vi "Read latest Position.vi"(8 "error in (no error)":errorcluster, 11 "FINE SIM Motion Axis":refnum<class "FINE SIM Motion Axis.lvclass">) -> (0 "error out":errorcluster, 2 "Current Position":dbl, 3 "FINE SIM Motion Axis":refnum<class "FINE SIM Motion Axis.lvclass">)   [LabVIEW 2022 SP3, in "FINE SIM Motion Axis.lvclass"]
uses:
  FINE SIM Motion Axis.lvclass
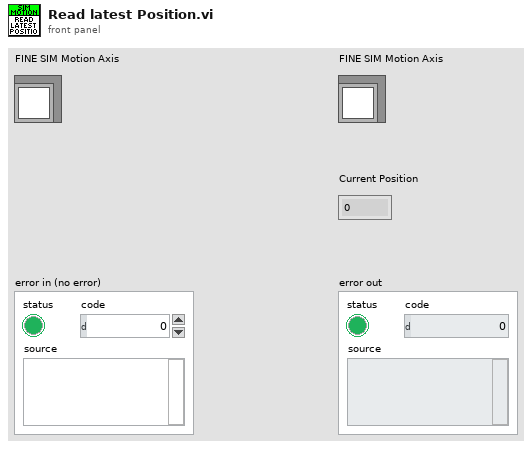
[diagram p1: front panel]
types:
  T1 = typedef "FINE SIM Motion Axis.lvclass/Axis Data.ctl" = cluster{"Axis Parameters":T2, "Time Stamp":timestamp, "Settings":T4}
  T2 = typedef "FINE SIM Motion Axis.lvclass/Axis Parameters.ctl" = cluster{"Moving":bool, "Homed":bool, "Desired Position":dbl, "Current Positon":dbl, "Current Speed":dbl, "Home Status":T3}
  T3 = typedef "FINE SIM Motion Axis.lvclass/Homing Status.ctl" = enum16{"Idle", "Inital Home Motion", "Final Home Motion", "Done Homing"}
  T4 = typedef "FINE SIM Motion Axis.lvclass/Settings.ctl" = cluster{"Axis Name":string, "Axis Settings":T5}
  T5 = typedef "FINE SIM Motion Axis.lvclass/Axis Settings.ctl" = cluster{"Speed":dbl, "Acceleration":dbl}
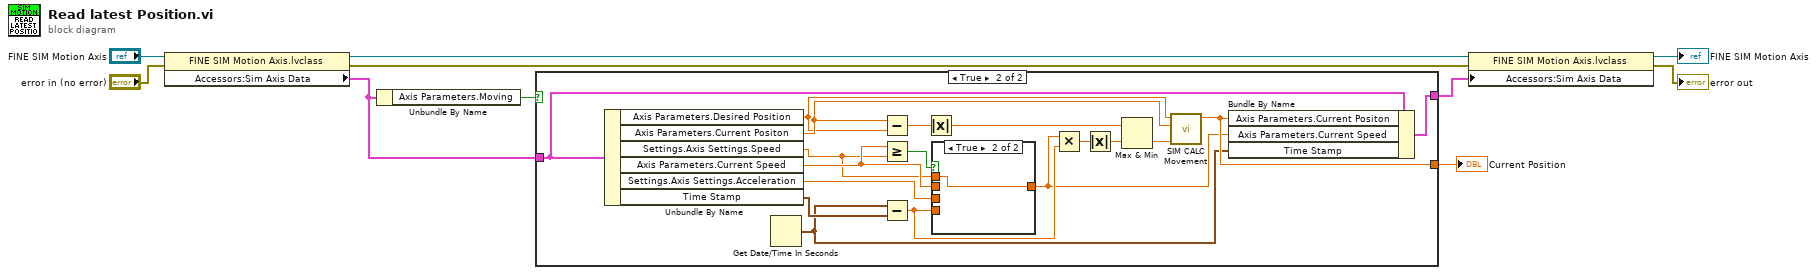
[diagram p0: block diagram]
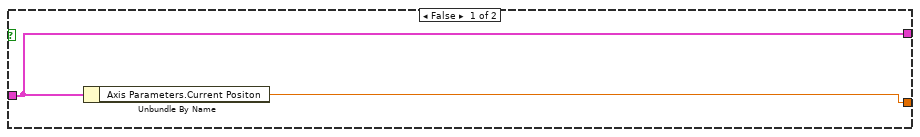
[diagram p2: hidden frame]
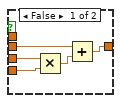
[diagram p3: hidden frame]
diagram:
  n1 = property class="FINE SIM Motion Axis.lvclass"(reference="FINE SIM Motion Axis", error in="error in (no error)") -> (reference out=w4:refnum<class "FINE SIM Motion Axis.lvclass">, error out=w7:errorcluster, "Accessors:Sim Axis Data"=w9:T1)
  n2 = Unbundle By Name(w9) -> ("Axis Parameters.Moving"=w8:bool)
  n3 = case shown="True" w8 {
    tunnel: w9 -> [w12 w30]
    tunnel: [w12 w28] -> w3
    tunnel: [w11 w29] -> w10
    frame False {
      n4 = Unbundle By Name(w12) -> ("Axis Parameters.Current Positon"=w11:dbl)
    }
    frame True {
      n5 = Unbundle By Name(w30) -> ("Axis Parameters.Desired Position"=w19:dbl, "Axis Parameters.Current Positon"=w20:dbl, "Settings.Axis Settings.Speed"=w13:dbl, "Axis Parameters.Current Speed"=w25:dbl, "Settings.Axis Settings.Acceleration"=w24:dbl, "Time Stamp"=w22:timestamp)
      n6 = Get Date/Time In Seconds() -> (seconds since 1Jan1904=w21:timestamp)
      n7 = Subtract(x=w20, y=w19) -> (x-y=w18:dbl)
      n8 = Greater Or Equal?(x=w25, y=w13) -> (x >= y?=w26:bool)
      n9 = Subtract(x=w21, y=w22) -> (x-y=w27:dbl)
      n10 = Absolute Value(x=w18) -> (abs(x)=w16:dbl)
      n11 = case shown="True" w26 {
        tunnel: [w31 w36] -> w23
        tunnel: w25 -> [w32 _]
        tunnel: w27 -> [w35 _]
        tunnel: w24 -> [w34 _]
        tunnel: w13 -> [_ w36]
        frame False {
          n12 = Multiply(x=w34, y=w35) -> (x*y=w33:dbl)
          n13 = Add(x=w32, y=w33) -> (x+y=w31:dbl)
        }
        frame True {
        }
      }
      n14 = Multiply(x=w23, y=w27) -> (x*y=w17:dbl)
      n15 = Absolute Value(x=w17) -> (abs(x)=w15:dbl)
      n16 = Max & Min(x=w16, y=w15) -> (min(x,y)=w14:dbl)  [unwired: 1 out]
      n17 = call "SIM CALC Movement.vi"("New Distance"=w14, "Current"=w20, "Desired"=w19) -> ("New Current"=w29:dbl)  [unwired: 8 in]
      n18 = Bundle By Name(cluster=w30, "Axis Parameters.Current Positon"=w29, "Axis Parameters.Current Speed"=w23, "Time Stamp"=w21) -> (w28:T1)
    }
  }
  "Current Position" <- w10
  n19 = property class="FINE SIM Motion Axis.lvclass"(reference=w4, error in=w7, "Accessors:Sim Axis Data"=w3) -> (reference out=→"FINE SIM Motion Axis":refnum<class "FINE SIM Motion Axis.lvclass">, error out=→"error out":errorcluster)
